vi "Fitness Core Override.vi"(8 "error in (no error)":errorcluster, 9 "Target Binary String (LSb[0] - MSb[n-1])":bool[](array[boolean]), 10 "Parent Binary String (LSb[0] - MSb[n-1])":bool[](array[boolean]), 11 "Solution in":refnum<class "Solution.lvclass">) -> (0 "error out":errorcluster, 2 "Fitness Score":dbl, 3 "Solution out":refnum<class "Solution.lvclass">)   [LabVIEW 2016, in "Solution.lvclass"]
uses:
  Solution.lvclass
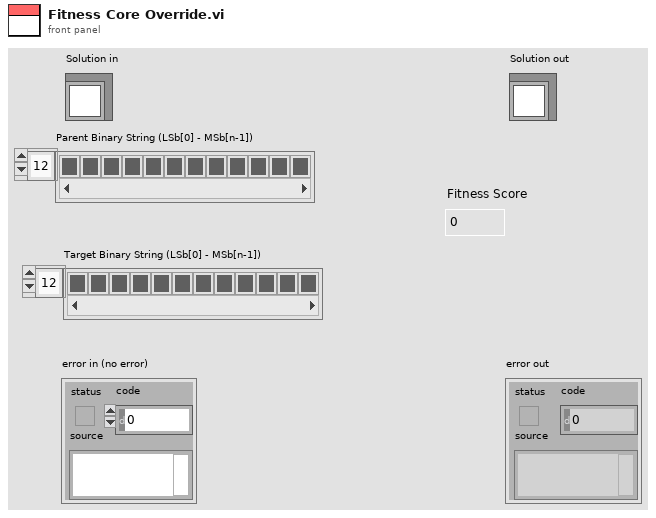
[diagram p1: front panel]
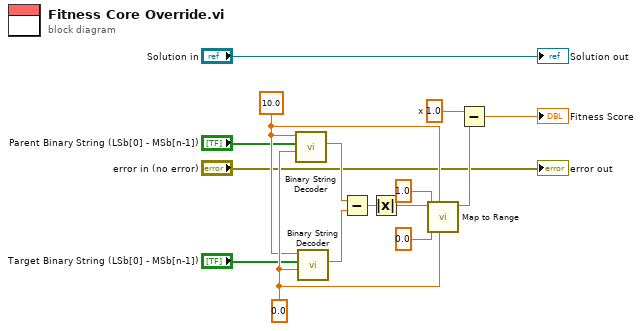
[diagram p0: block diagram]
diagram:
  w15 = 1.0  # x
  w11 = 0.0 ("X_L (0.0)")
  w10 = 10.0 ("X_U (1.0)")
  n1 = call "Binary String Decoder.vi"("X_L (0.0)"=w11, "Binary String (LSb[0] - MSb[n-1])"="Parent Binary String (LSb[0] - MSb[n-1])", "X_U (1.0)"=w10) -> ("x"=w6:dbl)  [unwired: 8 in]
  n2 = call "Binary String Decoder.vi"("X_L (0.0)"=w11, "Binary String (LSb[0] - MSb[n-1])"="Target Binary String (LSb[0] - MSb[n-1])", "X_U (1.0)"=w10) -> ("x"=w7:dbl)  [unwired: 8 in]
  n3 = Subtract(x=w6, y=w7) -> (x-y=w8:dbl)
  n4 = Absolute Value(x=w8) -> (abs(x)=w9:dbl)
  n5 = call "Map to Range.vi"("Value Min"=w11, "Value Max"=w10, "Scale Min"=0.0, "Scale Max"=1.0, "Value"=w9) -> ("Mapped Value"=w14:dbl)  [unwired: 6 in]
  n6 = Subtract(x=w15, y=w14) -> (x-y=→"Fitness Score":dbl)
  "error out" <- "error in (no error)"
  "Solution out" <- "Solution in"
